vi "FL Create Consequent.vi"(8 "error in (no error)":errorcluster, 10 "membership function index":i32, 11 "variable index":i32) -> (0 "error out":errorcluster, 3 "consequent":T1 {"Var Index" min=0; "Cond" items=["=", "!="]; "MF Index" min=0})   [LabVIEW 2013, in "NI_Fuzzy_Logic_API.lvlib"]
doc: "Creates a consequent, or THEN portion, of a rule for a fuzzy system. A consequent consists of three parts: an output linguistic variable, an operator that specifies to calculate the degree of membership of the output linguistic variable within a linguistic term, and a linguistic term.\n\nYou can use the Build Array function or a loop to build an array of rule consequents that you create with this VI. You then can wire the array to the <B>consequents</B> input of the FL Create Rule VI."
uses:
  <vilib>/addons/Fuzzy Logic/NI_Fuzzy_Logic_API.lvlib
  <vilib>/addons/Fuzzy Logic/TypeDefs/FL Consequent.ctl
  <vilib>/addons/Fuzzy Logic/TypeDefs/FL Modifier.ctl
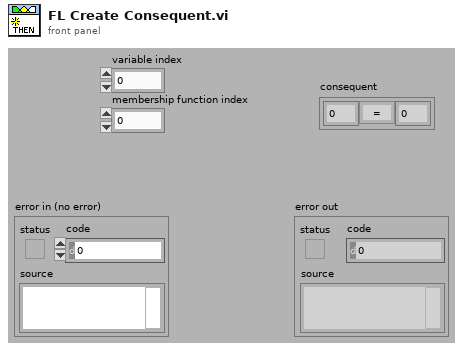
[diagram p1: front panel]
types:
  T1 = typedef "NI_Fuzzy_Logic_API.lvlib/FL Consequent.ctl" = cluster{"Var Index":i32, "MF Index":i32, "Cond":T2}
  T2 = typedef "NI_Fuzzy_Logic_API.lvlib/FL Modifier.ctl" = u16
  T3 = cluster{"variable index":i32, "membership function index":i32, "Cond":T2}
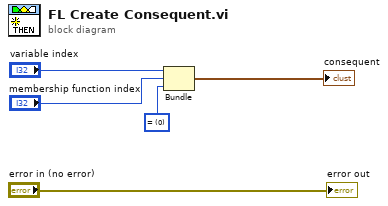
[diagram p0: block diagram]
diagram:
  w1 = T2 0 items=["=", "!="] ("Cond")
  n1 = Bundle("variable index"="variable index", "membership function index"="membership function index", "Cond"=w1) -> (→"consequent":T3)  [unwired: 1 out]
  "error out" <- "error in (no error)"
